vi "Archive Source File.vi"(8 "Error In":errorcluster, 10 "Source File":path, 11 "VIChallenge Config":T1={"AWS Credentials"={"AWSAccessKeyId"="", "Secret Key"=""}, "AWS Account Number"="", "SQS Jobs"=refnum, "SQS Status"=refnum, "Source Dir"=path "", "Working Dir"=path "", "Output Dir"=path "", "Archive Dir"=path "", "job"={"job_id"="", "challenge_id"="", "user_id"="", "s3_source_bucket"="", "s3_source_directory"="", "s3_source_filename"="", "status_queue_name"=""}, "Database Ref"=refnum, "Challenge Dir"=path "", "Challenges"=[]}) -> (0 "Error Out":errorcluster, 2 "Dup Source File":path, 3 "VIChallenge Config":T1)   [LabVIEW 2013, in "VIChallenge.lvlib"]
uses:
  VIChallenge.lvlib
  Type Defs/VIChallenge Config.ctl
  <vilib>/National Instruments/NI Amazon Web Services (AWS) Toolkit for LabVIEW/SQS/VI Source/AWS SQS Class/AWS_SQS.lvclass
  <vilib>/National Instruments/NI Amazon Web Services (AWS) Toolkit for LabVIEW/AWS Core Lib/VI Source/Canonicals/AWS_Core Canonical Credentials/Canonical Credentials.lvclass
  <vilib>/National Instruments/NI Amazon Web Services (AWS) Toolkit for LabVIEW/AWS Core Lib/VI Source/Canonicals/AWS_Core Canonical Required Parameters/Canonical Required Parameters.lvclass
  <vilib>/National Instruments/NI Amazon Web Services (AWS) Toolkit for LabVIEW/SQS/VI Source/Canonicals/Canonical CreateQueue/Canonical CreateQueue.lvclass
  <vilib>/National Instruments/NI Amazon Web Services (AWS) Toolkit for LabVIEW/SQS/VI Source/Canonicals/Canonical ListQueues/Canonical ListQueues.lvclass
  <vilib>/National Instruments/NI Amazon Web Services (AWS) Toolkit for LabVIEW/SQS/VI Source/Canonicals/Canonical AddPermission/Canonical AddPermission.lvclass
  <vilib>/National Instruments/NI Amazon Web Services (AWS) Toolkit for LabVIEW/SQS/VI Source/Canonicals/Canonical ChangeMessageVisibility/Canonical ChangeMessageVisibility.lvclass
  <vilib>/National Instruments/NI Amazon Web Services (AWS) Toolkit for LabVIEW/SQS/VI Source/Canonicals/Canonical ChangeMessageVisibilityBatch/Canonical ChangeMessageVisibilityBatch.lvclass
  <vilib>/National Instruments/NI Amazon Web Services (AWS) Toolkit for LabVIEW/SQS/VI Source/Canonicals/Canonical DeleteMessage/Canonical DeleteMessage.lvclass
  <vilib>/National Instruments/NI Amazon Web Services (AWS) Toolkit for LabVIEW/SQS/VI Source/Canonicals/Canonical DeleteMessageBatch/Canonical DeleteMessageBatch.lvclass
  <vilib>/National Instruments/NI Amazon Web Services (AWS) Toolkit for LabVIEW/SQS/VI Source/Canonicals/Canonical GetQueueAttributes/Canonical GetQueueAttributes.lvclass
  <vilib>/National Instruments/NI Amazon Web Services (AWS) Toolkit for LabVIEW/SQS/VI Source/Canonicals/Canonical GetQueueUrl/Canonical GetQueueUrl.lvclass
  <vilib>/National Instruments/NI Amazon Web Services (AWS) Toolkit for LabVIEW/SQS/VI Source/Canonicals/Canonical ReceiveMessage/Canonical ReceiveMessage.lvclass
  <vilib>/National Instruments/NI Amazon Web Services (AWS) Toolkit for LabVIEW/SQS/VI Source/Canonicals/Canonical RemovePermission/Canonical RemovePermission.lvclass
  <vilib>/National Instruments/NI Amazon Web Services (AWS) Toolkit for LabVIEW/SQS/VI Source/Canonicals/Canonical SendMessage/Canonical SendMessage.lvclass
  <vilib>/National Instruments/NI Amazon Web Services (AWS) Toolkit for LabVIEW/SQS/VI Source/Canonicals/Canonical SendMessageBatch/Canonical SendMessageBatch.lvclass
  <vilib>/National Instruments/NI Amazon Web Services (AWS) Toolkit for LabVIEW/SQS/VI Source/Canonicals/Canonical SetQueueAttributes/Canonical SetQueueAttributes.lvclass
  <vilib>/National Instruments/NI Amazon Web Services (AWS) Toolkit for LabVIEW/AWS Core Lib/VI Source/Typedefs/AWS_AWS Credentials.ctl
  Type Defs/JSON_job.ctl
  <vilib>/addons/database/Connection.llb/Conn ObjectReference.ctl
  Type Defs/Challenge.ctl
  <vilib>/National Instruments/NI Amazon Web Services (AWS) Toolkit for LabVIEW/AWS Core Lib/VI Source/AWS_Core.lvlib
  <vilib>/addons/database/NI_Database_API.lvlib
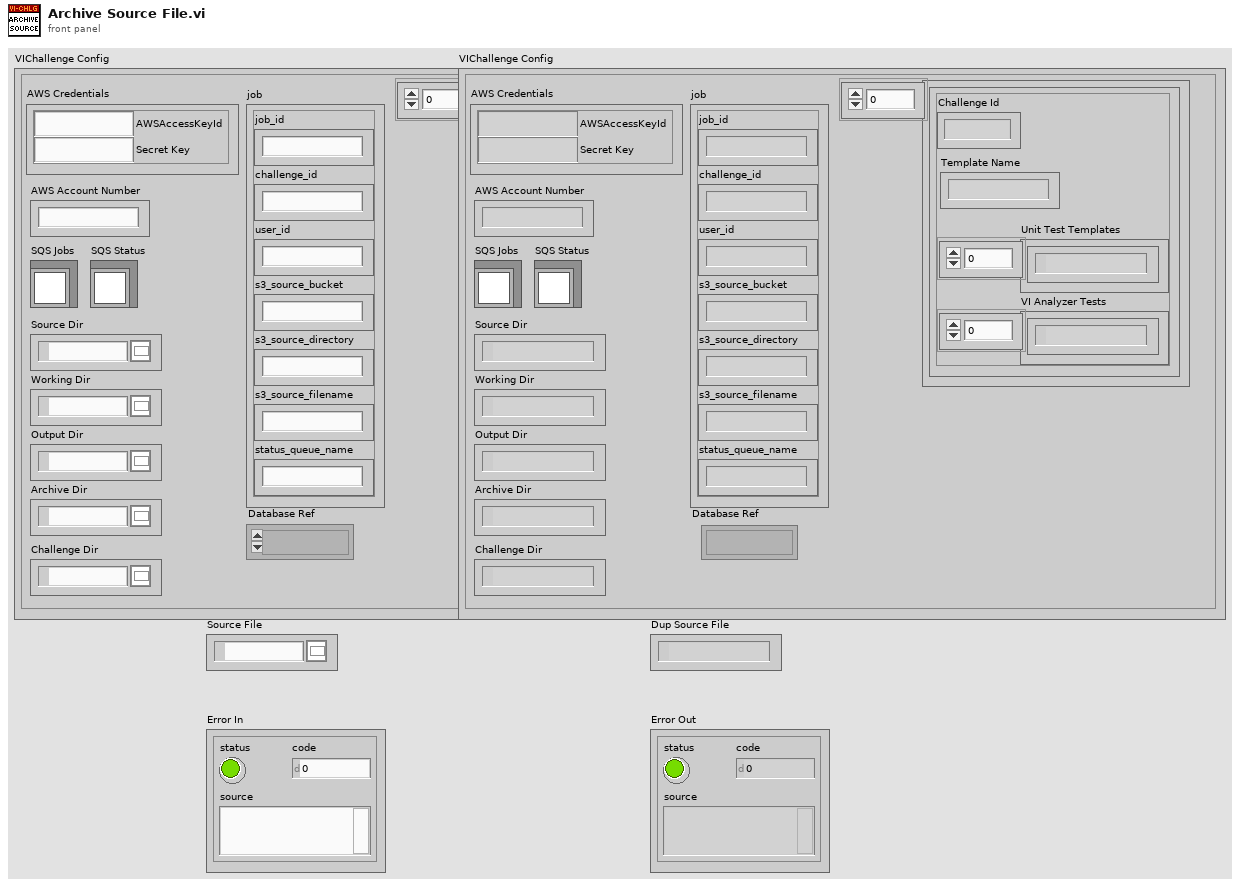
[diagram p1: front panel]
types:
  T1 = typedef "VIChallenge.lvlib/VIChallenge Config.ctl" = cluster{"AWS Credentials":T2, "AWS Account Number":string, "SQS Jobs":refnum<class "AWS_SQS.lvclass">, "SQS Status":refnum<class "AWS_SQS.lvclass">, "Source Dir":path, "Working Dir":path, "Output Dir":path, "Archive Dir":path, "job":T3, "Database Ref":T4, "Challenge Dir":path, "Challenges":T5[]}
  T2 = typedef "AWS_Core.lvlib/AWS_AWS Credentials.ctl" = cluster{"AWSAccessKeyId":string, "Secret Key":string}
  T3 = typedef "VIChallenge.lvlib/JSON_job.ctl" = cluster{"job_id":string, "challenge_id":string, "user_id":string, "s3_source_bucket":string, "s3_source_directory":string, "s3_source_filename":string, "status_queue_name":string}
  T4 = typedef "NI_Database_API.lvlib/Conn ObjectReference.ctl" = refnum<k1>
  T5 = typedef "VIChallenge.lvlib/Challenge.ctl" = cluster{"Challenge Id":i32, "Unit Test Templates":path[], "VI Analyzer Tests":path[], "Template Name":string}
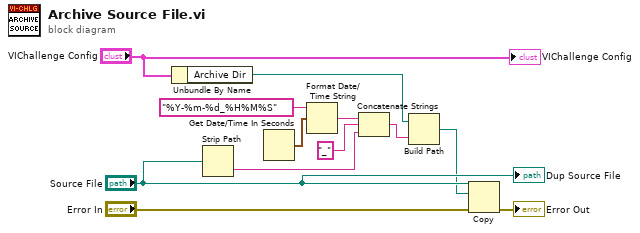
[diagram p0: block diagram]
diagram:
  n1 = Unbundle By Name("VIChallenge Config") -> ("Archive Dir"=w6:path)
  n2 = Strip Path(path="Source File") -> (name=w8:string)  [unwired: 1 out]
  n3 = Get Date/Time In Seconds() -> (seconds since 1Jan1904=w11:timestamp)
  n4 = Format Date/Time String(time format string (%c)="%Y-%m-%d_%H%M%S", seconds (now)=w11) -> (date/time string=w10:string)  [unwired: 1 in]
  n5 = Concatenate Strings(w10, "_" ("string"), w8) -> (w5:string)
  n6 = Build Path(base path=w6, name or relative path=w5) -> (appended path=w4:path)
  n7 = Copy(8:"Error In", 10:w4, 11:"Source File") -> (0:→"Error Out":errorcluster)  [unwired: 2 in, 2 out]
  "Dup Source File" <- "Source File"
  "VIChallenge Config" <- "VIChallenge Config"
